vi "ODE-VI-04022016.vi"(0 "Param_Value":dbl[](array[numeric])=[0.35, 180.0, 0.3], 1 "Mod_Value":dbl[](array[numeric]), 3 "Param_IDs":string[](array[string])=["k1", "k2", "compartment"], 4 "Mod_IDs":string[](array[string]), 5 "Initial Conditions for  variables":dbl[](array[numeric])=[0.00015, 0.0], 6 "Simulation Parameters":T4={"Initial Time"=0.0, "Final Time"=100.0, "Time Step"=0.1, "Absolute Tolerance"=0.001, "Relative Tolerance"=1e-06, "Type of Continuous Solver"=enum."Runge-Kutta 45 (variable)", "Discrete Time Step"=2.0, "Minimum Time Step"=1e-06, "Maximum Time Step"=1.0, "Initial Time Step"=0.1} {"Initial Time Step" min=0.0; "Maximum Time Step" min=0.0; "Minimum Time Step" min=0.0; "Discrete Time Step" min=0.0; "Relative Tolerance" min=0.0; "Absolute Tolerance" min=0.0; "Time Step" min=0.0}, 7 "ODE Right Hand Side":string[](array[string])=["-(compartment*k1*a0)+(compartment*k2*a1^2)", "-2*(compartment*k2*a1^2)+2*(compartment*k1*a0)"], 9 "Del Events":bool, 10 "Event Info":T3, 11 "X (name of variables)":string[](array[string])=["a0", "a1"], 12 "All Variables":string[](array[string]), 13 "Rest_Sp_Init_Amnt":string[](array[string])) -> (14 "Concentration vs. Time":cluster{"times":dbl[], dbl[]}[](graph), 19 "Sim Data":cluster{"times":dbl[], "outputs":dbl[][]} {"outputs" format="%#.9g"})   [LabVIEW 2014]
doc: "This example demonstrates how to use the polymorphic ODE solver in both Formula Sting mode and VI mode. Note that VI mode allows the user to set the values of constants via front panel controls, and the formula is implemented as a call by reference to another VI."
uses:
  ODE Simulation Parameters.ctl
  <vilib>/Simulation/Implementation/Shared/SIM Continuous Solvers.ctl
  Event Info.ctl
  <vilib>/Simulation/Utility/Implementation/Shared/SIM Diagram Parameters.ctl
  Stop ODE.vi
  <vilib>/gmath/ode.llb/ODE Solver formula string.vi
  Sim status.vi
  <vilib>/gmath/NI_Gmath.lvlib
panel:
  out "simulation parameters":T1={"Initial Time"=0.0, "Final Time"=10.0, "Time Step"=0.1, "Absolute Tolerance"=0.001, "Relative Tolerance"=0.001, "Continuous Solver"=enum."Runge-Kutta 45 (variable)", "Discrete Time Step"=1.0, "Minimum Time Step"=1e-08, "Maximum Time Step"=1.0, "Initial Time Step"=0.01} {"Initial Time Step" min=0.0; "Maximum Time Step" min=0.0}
  out "error out":errorcluster
  out "transposed array 2":dbl[][](array[numeric])
  out "subarray 2":dbl[](array[numeric])
  out "Array":dbl[][](array[numeric])
  out "transposed array":dbl[][](array[numeric])
  out "Assign Val":string[][](array[string])
  out "Assign Var Idx":i32[][](array[numeric])
  out "Var Idx":i32[](array[numeric])
  out "Math Val":string[](array[string])
  out "Math Op":string[](array[string])
  out "outputs":dbl[][](array[numeric])
  out "subarray":dbl[][](array[numeric])
  out "Flag":i32[](array[numeric])
  out "Delay Val Tot":dbl[](array[numeric])
  out "Delay Val":dbl[](array[numeric])
  out "Delay Val":dbl
  out "Priority":dbl[](array[numeric])
  out "Event Idx":i32
  out "Delay":dbl[](array[numeric])
  out "Total Mods":i32
  out "Time":dbl[](array[numeric])
  out "current data size":i32[](array[numeric])
  # "%"
  # "ds1/dt = - (k1*s1 - k2*s2) \nds2/dt = k1*s1 - k2*s2 - (s2*k2^nL/(k2^nL + s3^nL))\nds4/dt = s2*k2^nL/(k2^nL + s3^nL)\nds5/dt = - (s5 * (krp^nRP/(krp^nRP + s4^nRP))*(kG^nG/ (kG^nG + s6^nG)) - k4*s7)\nds7/dt = (s5 * (krp^nRP/(krp^nRP + s4^nRP))*(kG^nG/ (kG^nG + s6^nG)) - k4*s7) - k4*s7\nds8/dt = k4*s7"
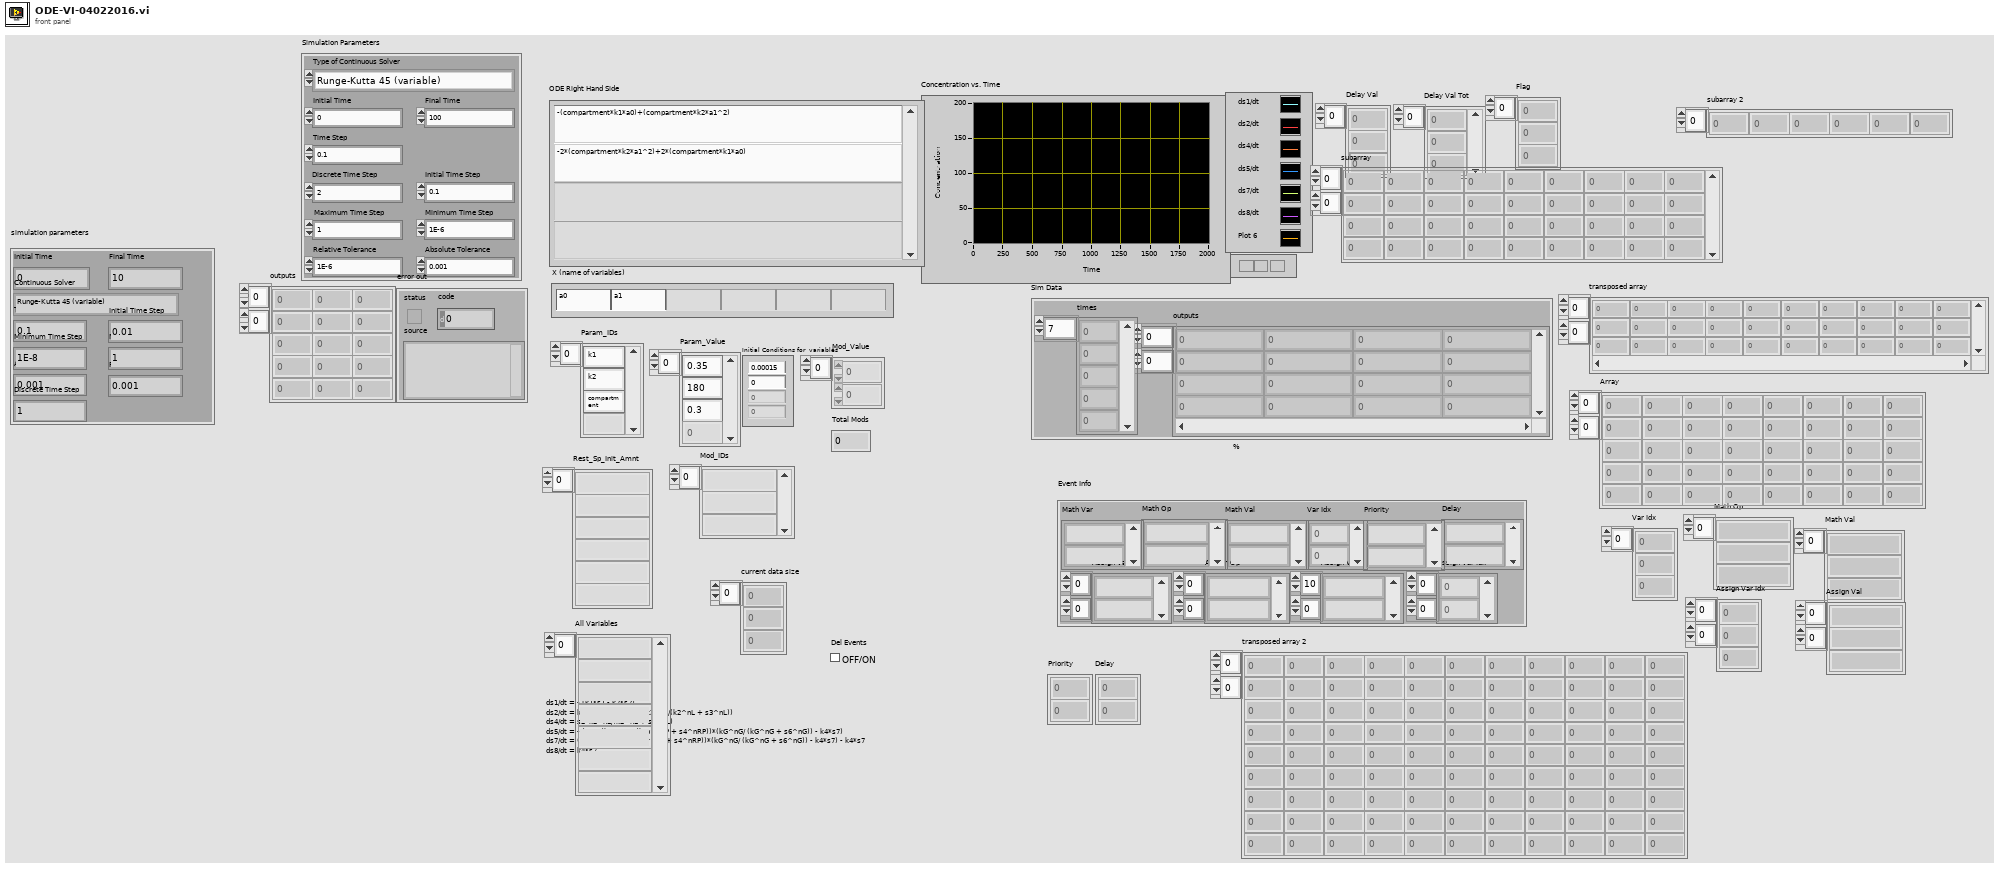
[diagram p1: front panel]
types:
  T1 = typedef "SIM Diagram Parameters.ctl" = cluster{"Initial Time":dbl, "Final Time":dbl, "Time Step":dbl, "Absolute Tolerance":dbl, "Relative Tolerance":dbl, "Continuous Solver":T2, "Discrete Time Step":dbl, "Minimum Time Step":dbl, "Maximum Time Step":dbl, "Initial Time Step":dbl}
  T2 = typedef "SIM Continuous Solvers.ctl" = enum16{"Runge-Kutta 1 (Euler)", "Runge-Kutta 2", "Runge-Kutta 3", "Runge-Kutta 4", "Runge-Kutta 23 (variable)", "Runge-Kutta 45 (variable)", "BDF (variable)", "Adams-Moulton (variable)", "Rosenbrock (variable)", "Discrete States Only"}
  T3 = typedef "Event Info.ctl" = cluster{"Math Var":string[], "Math Op":string[], "Math Val":string[], "Assign Var":string[][], "Assign Op":string[][], "Assign Val":string[][], "Var Idx":i32[], "Assign Var Idx":i32[][], "Delay":string[], "Priority":string[]}
  T4 = typedef "ODE Simulation Parameters.ctl" = cluster{"Initial Time":dbl, "Final Time":dbl, "Time Step":dbl, "Absolute Tolerance":dbl, "Relative Tolerance":dbl, "Type of Continuous Solver":T2, "Discrete Time Step":dbl, "Minimum Time Step":dbl, "Maximum Time Step":dbl, "Initial Time Step":dbl}
  T5 = cluster{"ODE Right Hand Side":string[], "X (name of variables)":string[], "time":string}
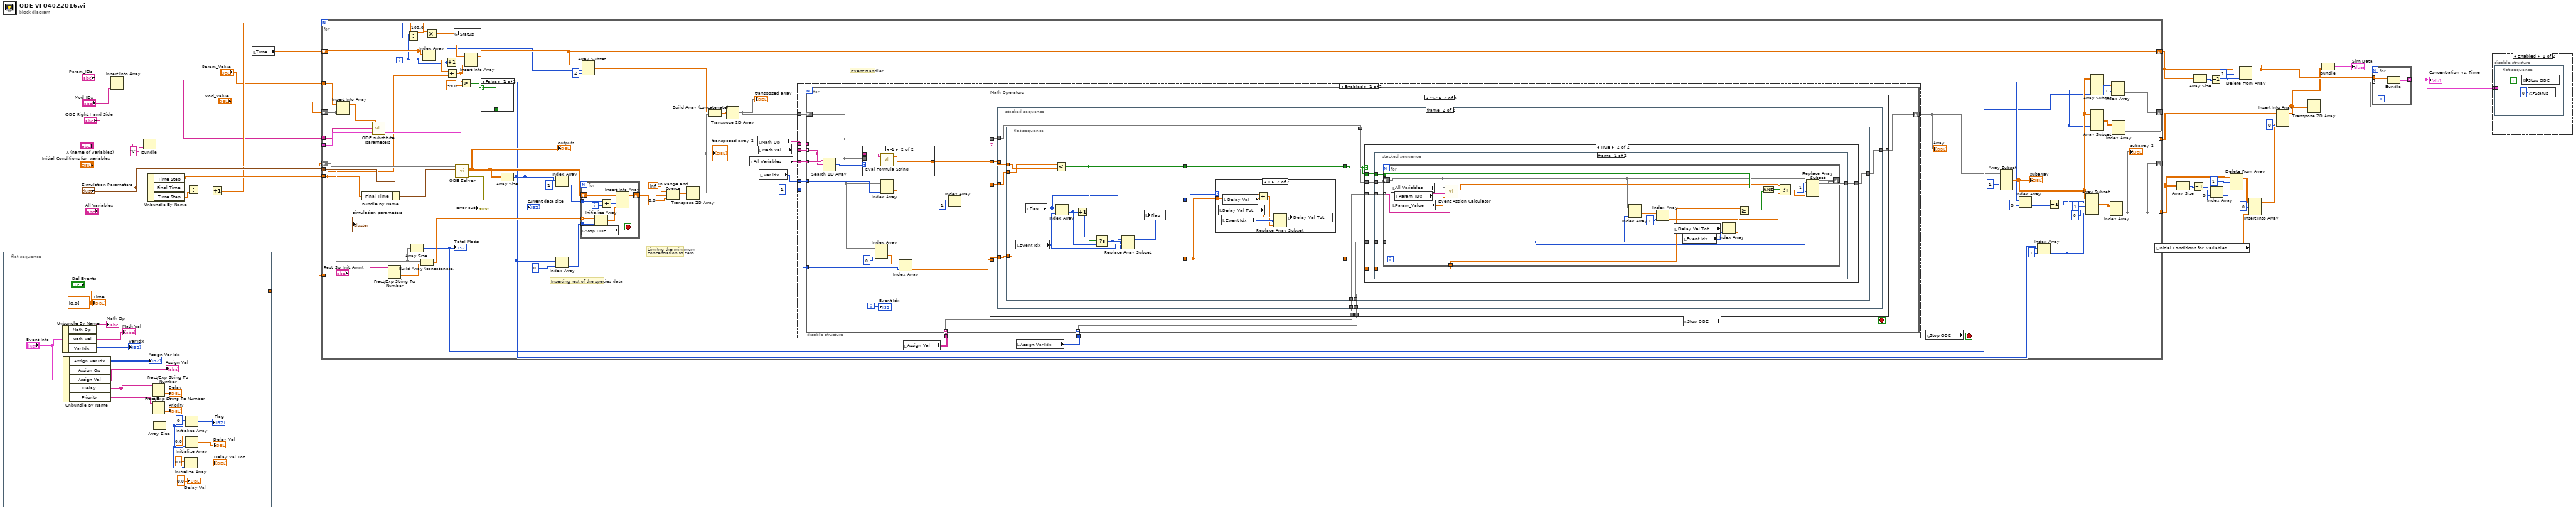
[diagram p0: block diagram]
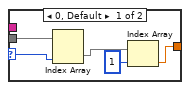
[diagram p4: hidden frame]
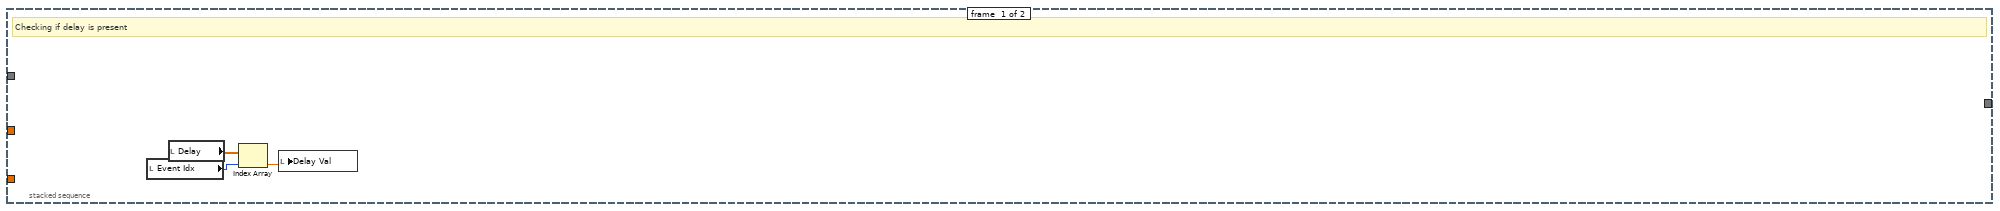
[diagram p6: hidden frame]
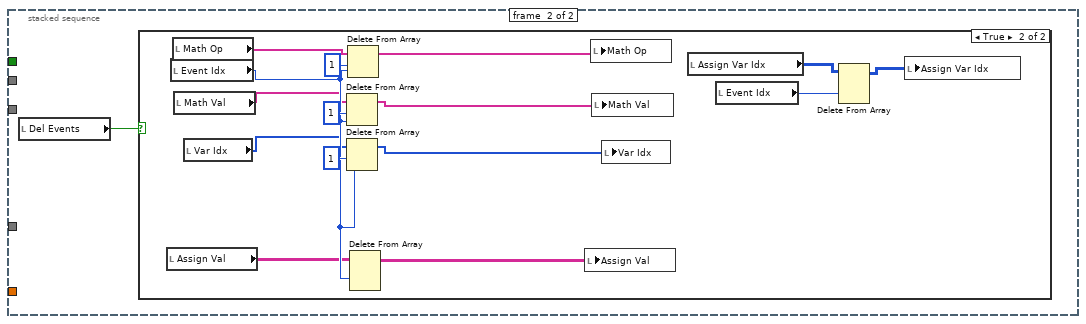
[diagram p9: hidden frame]
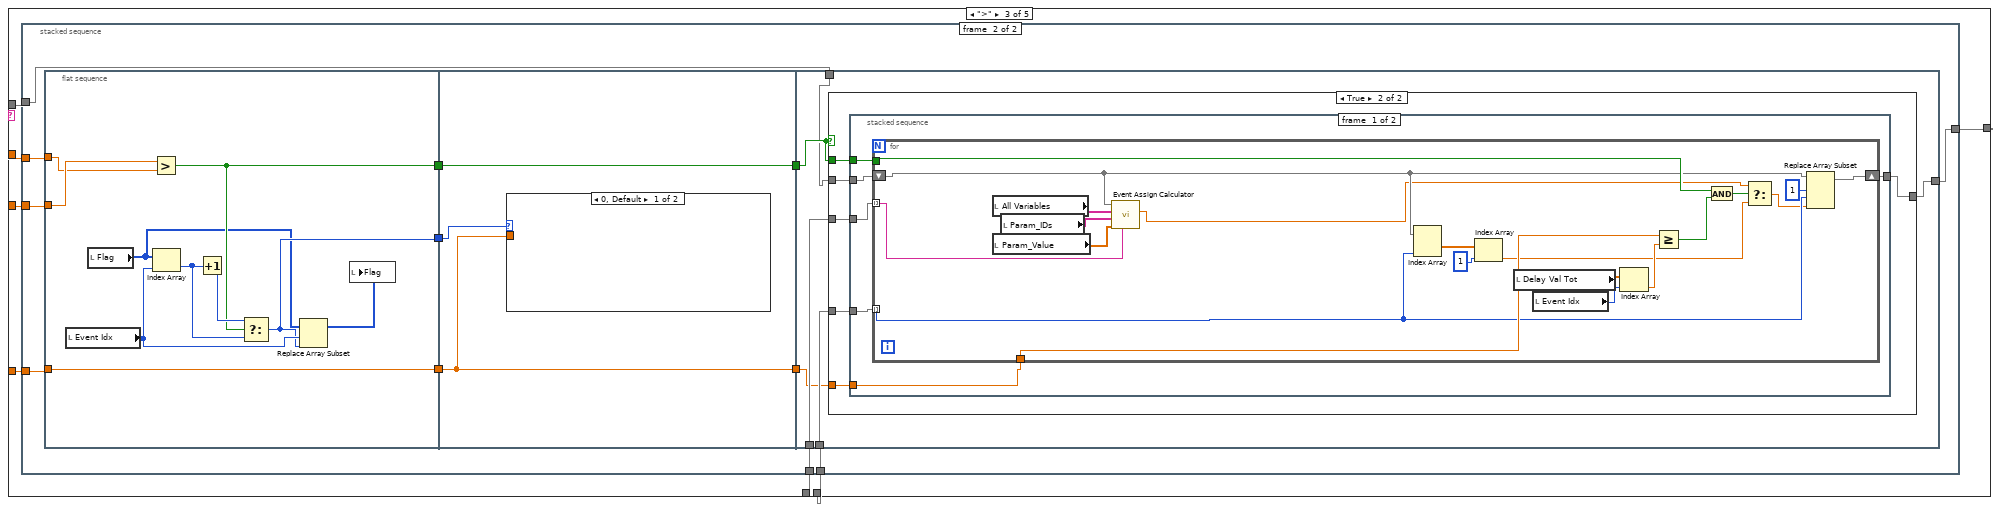
[diagram p11: hidden frame]
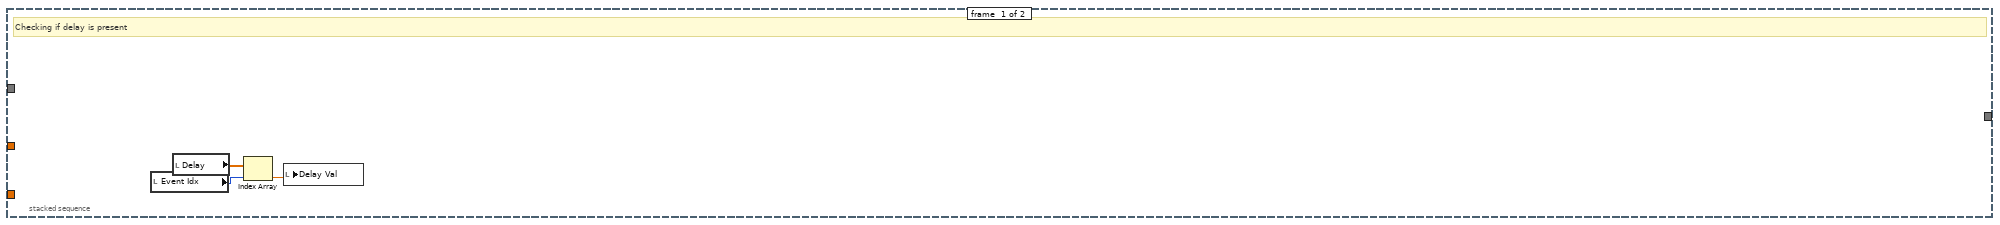
[diagram p12: hidden frame]
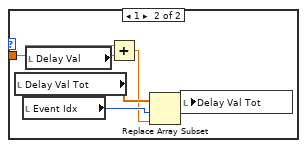
[diagram p13: hidden frame]
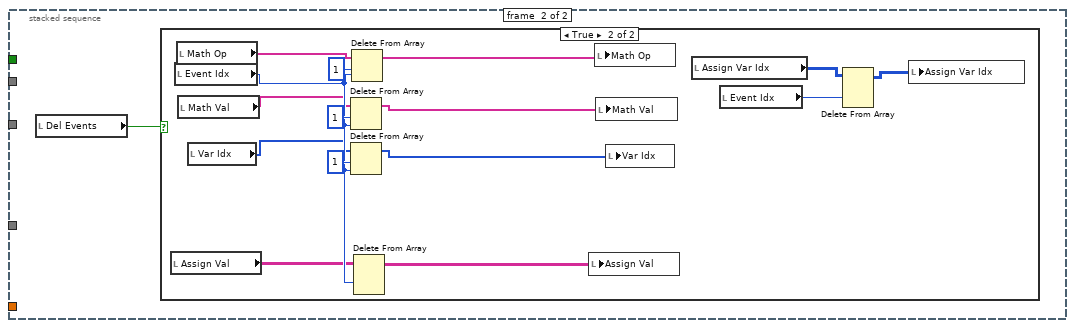
[diagram p15: hidden frame]
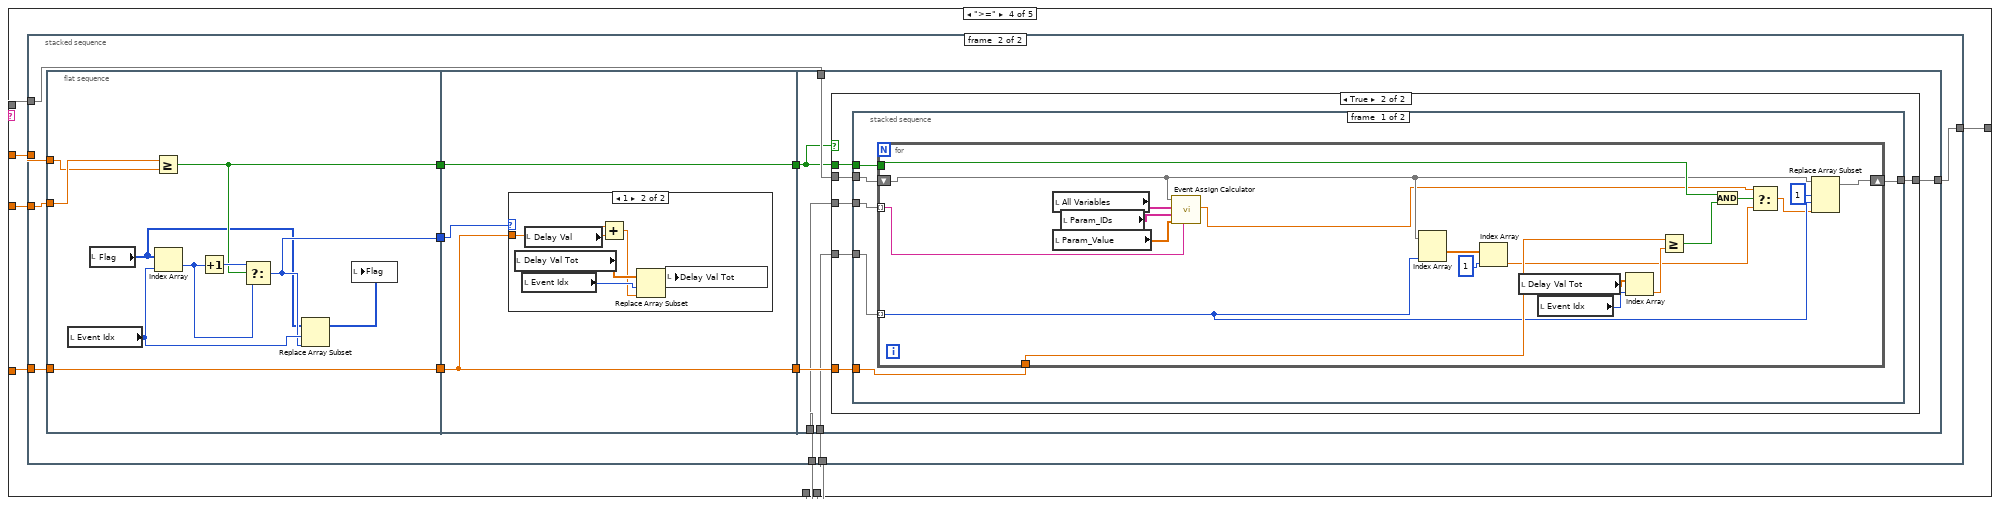
[diagram p17: hidden frame]
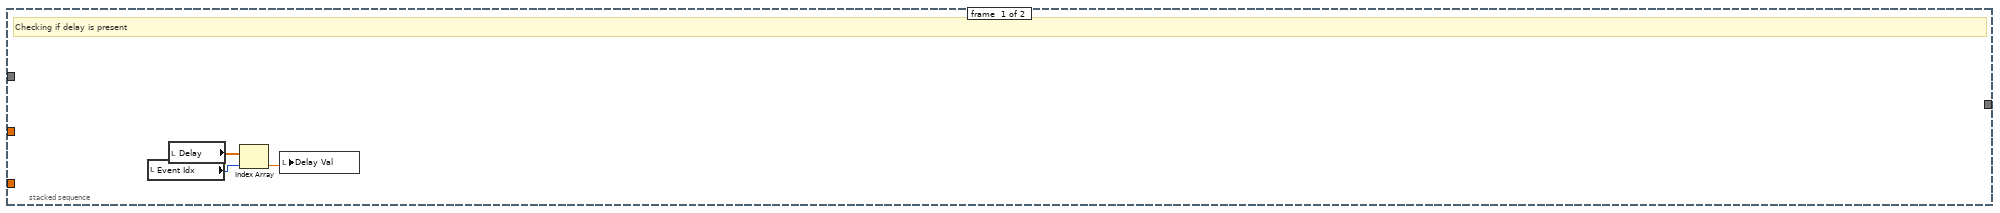
[diagram p18: hidden frame]
diagram:
  n1 = flat-sequence {
    tunnel: [w40] -> w1
    frame #0 {
      w40 = dbl[] [0.0]
      n2 = Unbundle By Name("Event Info") -> ("Math Op"=→"Math Op":string[], "Math Val"=→"Math Val":string[], "Var Idx"=→"Var Idx":i32[])
      n3 = Unbundle By Name("Event Info") -> ("Assign Var Idx"=→"Assign Var Idx":i32[][], "Assign Val"=→"Assign Val":string[][], "Delay"=w49:string[], "Priority"=w52:string[])  [unwired: 1 out]
      n4 = Fract/Exp String To Number(string=w49) -> (number=→"Delay":dbl[])  [unwired: 3 in, 1 out]
      n5 = Fract/Exp String To Number(string=w52) -> (number=→"Priority":dbl[])  [unwired: 3 in, 1 out]
      n6 = Array Size(array=w49) -> (size(s)=w44:i32)
      n7 = Initialize Array(0.0 ("element"), w44) -> (→"Delay Val Tot":dbl[])
      n8 = Initialize Array(0 ("element"), w44) -> (→"Flag":i32[])
      n9 = Initialize Array(0.0 ("element"), w44) -> (→"Delay Val":dbl[])
      "Time" <- w40
      "Delay Val" <- 0.0 ("Delay Val")
    }
  }
  n10 = Insert Into Array(array="Param_IDs", new element="Mod_IDs") -> (w5:string[])  [unwired: 1 in]
  n11 = Bundle("ODE Right Hand Side"="ODE Right Hand Side", "X (name of variables)"="X (name of variables)", "time"="t") -> (w6:T5)  [unwired: 1 in]
  n12 = Unbundle By Name("Simulation Parameters") -> ("Time Step"=w30:dbl, "Final Time"=w32:dbl, "Time Step"=w31:dbl)
  n13 = Divide(x=w32, y=w31) -> (x/y=w28:dbl)
  n14 = Increment(x=w28) -> (x+1=w27:dbl)
  n15 = local read "Time"() -> (w29:dbl[])
  n16 = for {
    N: w27 -> [w74]
    tunnel: "Simulation Parameters" -> [w104]
    shift-right: [w64] -> _
    shift-left: "Initial Conditions for  variables" -> [w125]
    shift-right: [w102] -> w25
    shift-left: w29 -> [w106]
    tunnel: [w64] -> w9 mode=indexing
    tunnel: w30 -> [w59]
    tunnel: [w97] -> w10 mode=indexing
    tunnel: w6 -> [w95]
    tunnel: w5 -> [w94]
    tunnel: "Param_Value" -> [w93]
    shift-right: [w77] -> _
    shift-left: "Mod_Value" -> [w89]
    tunnel: w1 -> [_]
    i -> [w75]
    stop <- w87 stop-if-true
    # "Event Handler"
    # "Limitng the minimum \nconcentration to zero"
    # "Inserting rest of the species data"
    n17 = Insert Into Array(array=w93, new element=w89) -> (w92:dbl[])  [unwired: 1 in]
    n18 = Bundle By Name(cluster=w104, "Final Time"=w59) -> (w103:T4)
    n19 = call "ODE substitute parameters.vi"("Formula String Parameters"=w95, "parameters"=w94, "values"=w92) -> ("Formula String Parameters with substitutions"=w96:T5)  [unwired: 2 out]
    n20 = Fract/Exp String To Number(string="Rest_Sp_Init_Amnt") -> (number=w118:dbl[])  [unwired: 3 in, 1 out]
    n21 = Divide(x=w75, y=w74) -> (x/y=w73:dbl)
    n22 = Array Size(array=w89) -> (size(s)=w88:i32)
    "Total Mods" <- w88
    n23 = Build Array (concatenate)(w89, w118) -> (w117:dbl[])
    n24 = Index Array(array=w106, index=w75) -> (element=w107:dbl)
    n25 = Multiply(x=100.0, y=w73) -> (x*y=w71:dbl)
    n26 = Increment(x=w75) -> (x+1=w105:i32)
    n27 = Add(x=w107, y=w59) -> (x+y=w81:dbl)
    n28 = global write "Sim status.vi" "Status"(w71) -> ()
    n29 = call-poly <vilib>:"ODE Solver.vi"("ODE RHS"=w96, "simulation parameters"=w103, "x0"=w125) -> ("error out"=→"error out":errorcluster, "outputs"=w120:dbl[][])  [unwired: 3 in, 4 out]
    "outputs" <- w120
    n30 = Greater Or Equal?(x=w81, y=99.0) -> (x >= y?=w79:bool)
    n31 = Insert Into Array(array=w106, index=w105, new element=w81) -> (w102:dbl[])
    n32 = case shown="False" w79 {
      selector: w79 -> [w126 w127]
      tunnel: [w126 w127] -> _
      frame False {
      }
      frame True {
      }
    }
    n33 = Array Size(array=w120) -> (size(s)=w99:i32[])
    "current data size" <- w99
    n34 = Index Array(array=w99, index=1) -> (element=w123:i32)
    n35 = Index Array(array=w99, index=0) -> (element=w121:i32)
    n36 = for {
      tunnel: w117 -> [w568] mode=indexing
      tunnel: w123 -> [w570]
      tunnel: w121 -> [w567]
      shift-right: [w564] -> w114
      shift-left: w120 -> [w565]
      i -> [w571]
      stop <- w563 stop-if-true
      n37 = global read "Stop ODE.vi" "Stop ODE"() -> (w563:bool)
      n38 = Initialize Array(w568, w567) -> (w566:dbl[])
      n39 = Add(x=w570, y=w571) -> (x+y=w569:i32)
      n40 = Insert Into Array(array=w565, index (col)=w569, new element=w566) -> (w564:dbl[][])  [unwired: 1 in]
    }
    n41 = Array Subset(array=w102, index=w75, length=2) -> (w100:dbl[])
    n42 = In Range and Coerce(upper limit=inf, x=w114, lower limit=0.0) -> (coerced(x)=w85:dbl[][])  [unwired: 1 out]
    n43 = Transpose 2D Array(2D array=w85) -> (transposed array=w84:dbl[][])
    "transposed array 2" <- w84
    n44 = Build Array (concatenate)(w100, w84) -> (w86:dbl[][])
    n45 = Transpose 2D Array(2D array=w86) -> (transposed array=w83:dbl[][])
    "transposed array" <- w83
    n46 = local read "All Variables"() -> (w65:string[])
    n47 = local read "Math Op"() -> (w70:string[])
    n48 = local read "Math Val"() -> (w69:string[])
    n49 = local read "Var Idx"() -> (w68:i32[])
    n50 = local read "Assign Val"() -> (w66:string[][])
    n51 = local read "Assign Var Idx"() -> (w67:i32[][])
    n52 = disable-structure shown="Enabled" {
      disable-tunnel: w70 -> [w136 w557]
      disable-tunnel: w69 -> [w135 w558]
      disable-tunnel: w68 -> [w134 w559]
      disable-tunnel: w66 -> [w129 w556]
      disable-tunnel: w67 -> [w133 w555]
      disable-tunnel: [w132 w561] -> w63
      disable-tunnel: w83 -> [w131 w562]
      disable-tunnel: 1 ("index") -> [w130 w560]
      disable-tunnel: w65 -> [w128 _]
      frame Enabled {
        n53 = for {
          tunnel: w136 -> [w155] mode=indexing
          tunnel: w135 -> [w139] mode=indexing
          tunnel: w134 -> [w154] mode=indexing
          tunnel: w129 -> [w150] mode=indexing
          tunnel: w133 -> [w153] mode=indexing
          shift-right: [w148] -> w132
          shift-left: w131 -> [w137]
          tunnel: w130 -> [w142]
          tunnel: w128 -> [w140]
          i -> [w151]
          stop <- w152 stop-if-true
          n54 = Search 1D Array(1D array=w140, element=w139) -> (index of element=w138:i32)  [unwired: 1 in]
          n55 = case shown="-1" w138 {
            selector: w138 -> [w159 _]
            tunnel: [w156 w161] -> w149
            tunnel: w139 -> [_ w162]
            tunnel: w137 -> [w160 _]
            frame 0, Default {
              n56 = Index Array(array=w160, index (col)=w159) -> (element=w157:dbl[])  [unwired: 1 in]
              n57 = Index Array(array=w157, index=1) -> (element=w156:dbl)
            }
            frame -1 {
              n58 = call <vilib>:"Eval Formula String.vi"("formula"=w162) -> ("y value"=w161:dbl)  [unwired: 1 in, 1 out]
            }
          }
          n59 = Index Array(array=w137, index (col)=0 ("disabled index (col)")) -> (element=w143:dbl[])  [unwired: 1 in]
          n60 = Index Array(array=w137, index (col)=w154) -> (element=w146:dbl[])  [unwired: 1 in]
          n61 = Index Array(array=w143, index=w142) -> (element=w141:dbl)
          n62 = Index Array(array=w146, index=1) -> (element=w145:dbl)
          n63 = case "Math Operators" shown="\"<\"" w155 {
            tunnel: w149 -> [_ w169 w265 w361 w457]
            tunnel: [w163 w168 w264 w360 w456] -> w148
            tunnel: w137 -> [w163 w170 w266 w362 w458]
            tunnel: w150 -> [_ w167 w263 w359 w455]
            tunnel: w153 -> [_ w166 w262 w358 w454]
            tunnel: w145 -> [_ w165 w261 w356 w453]
            tunnel: w141 -> [_ w164 w260 w357 w452]
            frame "False", Default {
            }
            frame "<" {
              n64 = stacked-sequence {
                tunnel: w169 -> [_ w185]
                tunnel: w170 -> [_ w177]
                tunnel: [_ w176] -> w168
                tunnel: w167 -> [_ w179]
                tunnel: w166 -> [_ w178]
                tunnel: w165 -> [_ w175]
                tunnel: w164 -> [_ w174]
                frame #0 {
                  # "Checking if delay is present"
                  n65 = local read "Event Idx"() -> (w172:i32)
                  n66 = local read "Delay"() -> (w173:dbl[])
                  n67 = Index Array(array=w173, index=w172) -> (element=w171:dbl)
                  n68 = local write "Delay Val"(w171) -> ()
                }
                frame #1 {
                  n69 = flat-sequence {
                    tunnel: w175 -> [w195]
                    tunnel: w185 -> [w194]
                    tunnel: [w189] -> w184
                    tunnel: [w188] -> w183
                    tunnel: [w186] -> w182
                    tunnel: w174 -> [w186]
                    tunnel: w184 -> [w197]
                    tunnel: w183 -> [w198]
                    tunnel: w182 -> [w196]
                    tunnel: [w198] -> w181
                    tunnel: [w196] -> w180
                    tunnel: w181 -> [w210]
                    tunnel: w180 -> [w206]
                    tunnel: w177 -> [w209]
                    tunnel: w178 -> [w207]
                    tunnel: w179 -> [w208]
                    tunnel: [w205] -> w176
                    frame #0 {
                      n70 = local read "Event Idx"() -> (w192:i32)
                      n71 = local read "Flag"() -> (w187:i32[])
                      n72 = Less?(x=w195, y=w194) -> (x < y?=w188:bool)
                      n73 = Index Array(array=w187, index=w192) -> (element=w191:i32)
                      n74 = Increment(x=w191) -> (x+1=w190:i32)
                      n75 = Select(t=w190, s=w188, f=w191) -> (s? t:f=w189:i32)
                      n76 = Replace Array Subset(array=w187, new element=w189, index=w192) -> (w193:i32[])
                      n77 = local write "Flag"(w193) -> ()
                    }
                    frame #1 {
                      n78 = case shown="1" w197 {
                        tunnel: w196 -> [_ w203]
                        frame 0, Default {
                        }
                        frame 1 {
                          n79 = local read "Delay Val Tot"() -> (w202:dbl[])
                          n80 = local read "Event Idx"() -> (w200:i32)
                          n81 = local read "Delay Val"() -> (w204:dbl)
                          n82 = Add(x=w203, y=w204) -> (x+y=w199:dbl)
                          n83 = Replace Array Subset(array=w202, new element=w199, index=w200) -> (w201:dbl[])
                          n84 = local write "Delay Val Tot"(w201) -> ()
                        }
                      }
                    }
                    frame #2 {
                      n85 = case shown="True" w210 {
                        tunnel: w210 -> [_ w217]
                        tunnel: w206 -> [_ w216]
                        tunnel: w209 -> [w211 w215]
                        tunnel: w207 -> [_ w214]
                        tunnel: w208 -> [_ w213]
                        tunnel: [w211 w212] -> w205
                        frame False {
                        }
                        frame True {
                          n86 = stacked-sequence {
                            tunnel: w217 -> [w223 _]
                            tunnel: w216 -> [w222 _]
                            tunnel: w215 -> [w221 _]
                            tunnel: w214 -> [w220 _]
                            tunnel: w213 -> [w219 _]
                            tunnel: [w218 _] -> w212
                            frame #0 {
                              n87 = for {
                                tunnel: w223 -> [w241]
                                tunnel: w222 -> [w240]
                                tunnel: w220 -> [w232] mode=indexing
                                tunnel: w219 -> [w225] mode=indexing
                                shift-right: [w230] -> w218
                                shift-left: w221 -> [w229]
                                n88 = local read "All Variables"() -> (w228:string[])
                                n89 = local read "Param_Value"() -> (w226:dbl[])
                                n90 = local read "Param_IDs"() -> (w227:string[])
                                n91 = call "Event Assign Calculator.vi"("Assign Val"=w225, "Param_Value"=w226, "Param_IDs"=w227, "All Variables"=w228, "transposed array"=w229) -> ("y value"=w224:dbl)  [unwired: 6 in]
                                n92 = Index Array(array=w229, index (col)=w232) -> (element=w235:dbl[])  [unwired: 1 in]
                                n93 = Index Array(array=w235, index=1) -> (element=w234:dbl)
                                n94 = local read "Delay Val Tot"() -> (w239:dbl[])
                                n95 = local read "Event Idx"() -> (w238:i32)
                                n96 = Index Array(array=w239, index=w238) -> (element=w237:dbl)
                                n97 = Greater Or Equal?(x=w240, y=w237) -> (x >= y?=w242:bool)
                                n98 = And(x=w241, y=w242) -> (x .and. y?=w243:bool)
                                n99 = Select(t=w224, s=w243, f=w234) -> (s? t:f=w231:dbl)
                                n100 = Replace Array Subset(array=w229, new element=w231, index (row)=1, index (col)=w232) -> (w230:dbl[][])
                              }
                            }
                            frame #1 {
                              n101 = local read "Del Events"() -> (w244:bool)
                              n102 = case shown="True" w244 {
                                frame False {
                                }
                                frame True {
                                n103 = local read "Assign Val"() -> (w249:string[][])
                                n104 = local read "Event Idx"() -> (w256:i32)
                                n105 = local read "Math Op"() -> (w255:string[])
                                n106 = local read "Math Val"() -> (w254:string[])
                                n107 = local read "Var Idx"() -> (w253:i32[])
                                n108 = Delete From Array(array=w254, length=1, index=w256) -> (array with subset deleted=w251:string[])  [unwired: 1 out]
                                n109 = Delete From Array(array=w253, length=1, index=w256) -> (array with subset deleted=w250:i32[])  [unwired: 1 out]
                                n110 = Delete From Array(array=w255, length=1, index=w256) -> (array with subset deleted=w252:string[])  [unwired: 1 out]
                                n111 = Delete From Array(array=w249, index (row)=w256) -> (array with subset deleted=w248:string[][])  [unwired: 2 in, 1 out]
                                n112 = local write "Assign Val"(w248) -> ()
                                n113 = local write "Math Op"(w252) -> ()
                                n114 = local write "Math Val"(w251) -> ()
                                n115 = local write "Var Idx"(w250) -> ()
                                n116 = local read "Assign Var Idx"() -> (w247:i32[][])
                                n117 = local read "Event Idx"() -> (w246:i32)
                                n118 = Delete From Array(array=w247, index (row)=w246) -> (array with subset deleted=w245:i32[][])  [unwired: 2 in, 1 out]
                                n119 = local write "Assign Var Idx"(w245) -> ()
                                }
                              }
                            }
                          }
                        }
                      }
                    }
                  }
                }
              }
            }
            frame ">" {
              n120 = stacked-sequence {
                tunnel: w265 -> [_ w281]
                tunnel: w266 -> [_ w273]
                tunnel: [_ w272] -> w264
                tunnel: w263 -> [_ w275]
                tunnel: w262 -> [_ w274]
                tunnel: w261 -> [_ w271]
                tunnel: w260 -> [_ w270]
                frame #0 {
                  # "Checking if delay is present"
                  n121 = local read "Event Idx"() -> (w268:i32)
                  n122 = local read "Delay"() -> (w269:dbl[])
                  n123 = Index Array(array=w269, index=w268) -> (element=w267:dbl)
                  n124 = local write "Delay Val"(w267) -> ()
                }
                frame #1 {
                  n125 = flat-sequence {
                    tunnel: w271 -> [w291]
                    tunnel: w281 -> [w290]
                    tunnel: w270 -> [w289]
                    tunnel: [w284] -> w280
                    tunnel: [w283] -> w279
                    tunnel: [w289] -> w278
                    tunnel: w280 -> [w293]
                    tunnel: w279 -> [w294]
                    tunnel: w278 -> [w292]
                    tunnel: [w294] -> w277
                    tunnel: [w292] -> w276
                    tunnel: w277 -> [w306]
                    tunnel: w276 -> [w302]
                    tunnel: w273 -> [w305]
                    tunnel: w274 -> [w303]
                    tunnel: w275 -> [w304]
                    tunnel: [w301] -> w272
                    frame #0 {
                      n126 = local read "Event Idx"() -> (w287:i32)
                      n127 = local read "Flag"() -> (w282:i32[])
                      n128 = Greater?(x=w291, y=w290) -> (0:w283:bool)
                      n129 = Index Array(array=w282, index=w287) -> (element=w286:i32)
                      n130 = Increment(x=w286) -> (x+1=w285:i32)
                      n131 = Select(t=w285, s=w283, f=w286) -> (s? t:f=w284:i32)
                      n132 = Replace Array Subset(array=w282, new element=w284, index=w287) -> (w288:i32[])
                      n133 = local write "Flag"(w288) -> ()
                    }
                    frame #1 {
                      n134 = case shown="0, Default" w293 {
                        tunnel: w292 -> [_ w299]
                        frame 0, Default {
                        }
                        frame 1 {
                          n135 = local read "Delay Val Tot"() -> (w298:dbl[])
                          n136 = local read "Event Idx"() -> (w296:i32)
                          n137 = local read "Delay Val"() -> (w300:dbl)
                          n138 = Add(x=w299, y=w300) -> (x+y=w295:dbl)
                          n139 = Replace Array Subset(array=w298, new element=w295, index=w296) -> (w297:dbl[])
                          n140 = local write "Delay Val Tot"(w297) -> ()
                        }
                      }
                    }
                    frame #2 {
                      n141 = case shown="True" w306 {
                        tunnel: w306 -> [_ w313]
                        tunnel: w302 -> [_ w312]
                        tunnel: w305 -> [w307 w311]
                        tunnel: w303 -> [_ w310]
                        tunnel: w304 -> [_ w309]
                        tunnel: [w307 w308] -> w301
                        frame False {
                        }
                        frame True {
                          n142 = stacked-sequence {
                            tunnel: w313 -> [w317 _]
                            tunnel: w312 -> [w314 _]
                            tunnel: w311 -> [w316 _]
                            tunnel: w310 -> [w318 _]
                            tunnel: w309 -> [w315 _]
                            tunnel: [w319 _] -> w308
                            frame #0 {
                              n143 = for {
                                tunnel: w317 -> [w337]
                                tunnel: w314 -> [w336]
                                tunnel: w318 -> [w328] mode=indexing
                                tunnel: w315 -> [w322] mode=indexing
                                shift-right: [w326] -> w319
                                shift-left: w316 -> [w321]
                                n144 = local read "All Variables"() -> (w325:string[])
                                n145 = local read "Param_Value"() -> (w323:dbl[])
                                n146 = local read "Param_IDs"() -> (w324:string[])
                                n147 = call "Event Assign Calculator.vi"("Assign Val"=w322, "Param_Value"=w323, "Param_IDs"=w324, "All Variables"=w325, "transposed array"=w321) -> ("y value"=w320:dbl)  [unwired: 6 in]
                                n148 = Index Array(array=w321, index (col)=w328) -> (element=w331:dbl[])  [unwired: 1 in]
                                n149 = Index Array(array=w331, index=1) -> (element=w330:dbl)
                                n150 = local read "Delay Val Tot"() -> (w335:dbl[])
                                n151 = local read "Event Idx"() -> (w334:i32)
                                n152 = Index Array(array=w335, index=w334) -> (element=w333:dbl)
                                n153 = Greater Or Equal?(x=w336, y=w333) -> (x >= y?=w338:bool)
                                n154 = And(x=w337, y=w338) -> (x .and. y?=w339:bool)
                                n155 = Select(t=w320, s=w339, f=w330) -> (s? t:f=w327:dbl)
                                n156 = Replace Array Subset(array=w321, new element=w327, index (row)=1, index (col)=w328) -> (w326:dbl[][])
                              }
                            }
                            frame #1 {
                              n157 = local read "Del Events"() -> (w340:bool)
                              n158 = case shown="True" w340 {
                                frame False {
                                }
                                frame True {
                                n159 = local read "Assign Val"() -> (w345:string[][])
                                n160 = local read "Event Idx"() -> (w352:i32)
                                n161 = local read "Math Op"() -> (w351:string[])
                                n162 = local read "Math Val"() -> (w350:string[])
                                n163 = local read "Var Idx"() -> (w349:i32[])
                                n164 = Delete From Array(array=w350, length=1, index=w352) -> (array with subset deleted=w347:string[])  [unwired: 1 out]
                                n165 = Delete From Array(array=w349, length=1, index=w352) -> (array with subset deleted=w346:i32[])  [unwired: 1 out]
                                n166 = Delete From Array(array=w351, length=1, index=w352) -> (array with subset deleted=w348:string[])  [unwired: 1 out]
                                n167 = Delete From Array(array=w345, index (row)=w352) -> (array with subset deleted=w344:string[][])  [unwired: 2 in, 1 out]
                                n168 = local write "Assign Val"(w344) -> ()
                                n169 = local write "Math Op"(w348) -> ()
                                n170 = local write "Math Val"(w347) -> ()
                                n171 = local write "Var Idx"(w346) -> ()
                                n172 = local read "Assign Var Idx"() -> (w343:i32[][])
                                n173 = local read "Event Idx"() -> (w342:i32)
                                n174 = Delete From Array(array=w343, index (row)=w342) -> (array with subset deleted=w341:i32[][])  [unwired: 2 in, 1 out]
                                n175 = local write "Assign Var Idx"(w341) -> ()
                                }
                              }
                            }
                          }
                        }
                      }
                    }
                  }
                }
              }
            }
            frame ">=" {
              n176 = stacked-sequence {
                tunnel: w361 -> [_ w377]
                tunnel: w362 -> [_ w369]
                tunnel: [_ w368] -> w360
                tunnel: w359 -> [_ w371]
                tunnel: w358 -> [_ w370]
                tunnel: w357 -> [_ w367]
                tunnel: w356 -> [_ w366]
                frame #0 {
                  # "Checking if delay is present"
                  n177 = local read "Event Idx"() -> (w364:i32)
                  n178 = local read "Delay"() -> (w365:dbl[])
                  n179 = Index Array(array=w365, index=w364) -> (element=w363:dbl)
                  n180 = local write "Delay Val"(w363) -> ()
                }
                frame #1 {
                  n181 = flat-sequence {
                    tunnel: w366 -> [w387]
                    tunnel: w377 -> [w386]
                    tunnel: w367 -> [w385]
                    tunnel: [w380] -> w376
                    tunnel: [w379] -> w375
                    tunnel: [w385] -> w374
                    tunnel: w376 -> [w389]
                    tunnel: w375 -> [w390]
                    tunnel: w374 -> [w388]
                    tunnel: [w390] -> w373
                    tunnel: [w388] -> w372
                    tunnel: w373 -> [w397]
                    tunnel: w372 -> [w402]
                    tunnel: w369 -> [w401]
                    tunnel: w370 -> [w400]
                    tunnel: w371 -> [w399]
                    tunnel: [w398] -> w368
                    frame #0 {
                      n182 = local read "Event Idx"() -> (w383:i32)
                      n183 = local read "Flag"() -> (w378:i32[])
                      n184 = Greater Or Equal?(x=w387, y=w386) -> (x >= y?=w379:bool)
                      n185 = Index Array(array=w378, index=w383) -> (element=w382:i32)
                      n186 = Increment(x=w382) -> (x+1=w381:i32)
                      n187 = Select(t=w381, s=w379, f=w382) -> (s? t:f=w380:i32)
                      n188 = Replace Array Subset(array=w378, new element=w380, index=w383) -> (w384:i32[])
                      n189 = local write "Flag"(w384) -> ()
                    }
                    frame #1 {
                      n190 = case shown="1" w389 {
                        tunnel: w388 -> [_ w395]
                        frame 0, Default {
                        }
                        frame 1 {
                          n191 = local read "Delay Val Tot"() -> (w394:dbl[])
                          n192 = local read "Event Idx"() -> (w392:i32)
                          n193 = local read "Delay Val"() -> (w396:dbl)
                          n194 = Add(x=w395, y=w396) -> (x+y=w391:dbl)
                          n195 = Replace Array Subset(array=w394, new element=w391, index=w392) -> (w393:dbl[])
                          n196 = local write "Delay Val Tot"(w393) -> ()
                        }
                      }
                    }
                    frame #2 {
                      n197 = case shown="True" w397 {
                        tunnel: w397 -> [_ w409]
                        tunnel: w402 -> [_ w408]
                        tunnel: w401 -> [w403 w407]
                        tunnel: w400 -> [_ w406]
                        tunnel: w399 -> [_ w405]
                        tunnel: [w403 w404] -> w398
                        frame False {
                        }
                        frame True {
                          n198 = stacked-sequence {
                            tunnel: w409 -> [w414 _]
                            tunnel: w408 -> [w411 _]
                            tunnel: w407 -> [w415 _]
                            tunnel: w406 -> [w412 _]
                            tunnel: w405 -> [w413 _]
                            tunnel: [w410 _] -> w404
                            frame #0 {
                              n199 = for {
                                tunnel: w414 -> [w433]
                                tunnel: w411 -> [w432]
                                tunnel: w412 -> [w424] mode=indexing
                                tunnel: w413 -> [w418] mode=indexing
                                shift-right: [w422] -> w410
                                shift-left: w415 -> [w417]
                                n200 = local read "All Variables"() -> (w421:string[])
                                n201 = local read "Param_Value"() -> (w419:dbl[])
                                n202 = local read "Param_IDs"() -> (w420:string[])
                                n203 = call "Event Assign Calculator.vi"("Assign Val"=w418, "Param_Value"=w419, "Param_IDs"=w420, "All Variables"=w421, "transposed array"=w417) -> ("y value"=w416:dbl)  [unwired: 6 in]
                                n204 = Index Array(array=w417, index (col)=w424) -> (element=w427:dbl[])  [unwired: 1 in]
                                n205 = Index Array(array=w427, index=1) -> (element=w426:dbl)
                                n206 = local read "Delay Val Tot"() -> (w431:dbl[])
                                n207 = local read "Event Idx"() -> (w430:i32)
                                n208 = Index Array(array=w431, index=w430) -> (element=w429:dbl)
                                n209 = Greater Or Equal?(x=w432, y=w429) -> (x >= y?=w434:bool)
                                n210 = And(x=w433, y=w434) -> (x .and. y?=w435:bool)
                                n211 = Select(t=w416, s=w435, f=w426) -> (s? t:f=w423:dbl)
                                n212 = Replace Array Subset(array=w417, new element=w423, index (row)=1, index (col)=w424) -> (w422:dbl[][])
                              }
                            }
                            frame #1 {
                              n213 = local read "Del Events"() -> (w436:bool)
                              n214 = case shown="True" w436 {
                                frame False {
                                }
                                frame True {
                                n215 = local read "Assign Val"() -> (w441:string[][])
                                n216 = local read "Event Idx"() -> (w448:i32)
                                n217 = local read "Math Op"() -> (w447:string[])
                                n218 = local read "Math Val"() -> (w446:string[])
                                n219 = local read "Var Idx"() -> (w445:i32[])
                                n220 = Delete From Array(array=w446, length=1, index=w448) -> (array with subset deleted=w443:string[])  [unwired: 1 out]
                                n221 = Delete From Array(array=w445, length=1, index=w448) -> (array with subset deleted=w442:i32[])  [unwired: 1 out]
                                n222 = Delete From Array(array=w447, length=1, index=w448) -> (array with subset deleted=w444:string[])  [unwired: 1 out]
                                n223 = Delete From Array(array=w441, index (row)=w448) -> (array with subset deleted=w440:string[][])  [unwired: 2 in, 1 out]
                                n224 = local write "Assign Val"(w440) -> ()
                                n225 = local write "Math Op"(w444) -> ()
                                n226 = local write "Math Val"(w443) -> ()
                                n227 = local write "Var Idx"(w442) -> ()
                                n228 = local read "Assign Var Idx"() -> (w439:i32[][])
                                n229 = local read "Event Idx"() -> (w438:i32)
                                n230 = Delete From Array(array=w439, index (row)=w438) -> (array with subset deleted=w437:i32[][])  [unwired: 2 in, 1 out]
                                n231 = local write "Assign Var Idx"(w437) -> ()
                                }
                              }
                            }
                          }
                        }
                      }
                    }
                  }
                }
              }
            }
            frame "<=" {
              n232 = stacked-sequence {
                tunnel: w457 -> [_ w473]
                tunnel: w458 -> [_ w465]
                tunnel: [_ w462] -> w456
                tunnel: w455 -> [_ w467]
                tunnel: w454 -> [_ w466]
                tunnel: w453 -> [_ w464]
                tunnel: w452 -> [_ w463]
                frame #0 {
                  # "Checking if delay is present"
                  n233 = local read "Event Idx"() -> (w460:i32)
                  n234 = local read "Delay"() -> (w461:dbl[])
                  n235 = Index Array(array=w461, index=w460) -> (element=w459:dbl)
                  n236 = local write "Delay Val"(w459) -> ()
                }
                frame #1 {
                  n237 = flat-sequence {
                    tunnel: w464 -> [w483]
                    tunnel: w473 -> [w482]
                    tunnel: w463 -> [w481]
                    tunnel: [w476] -> w472
                    tunnel: [w475] -> w471
                    tunnel: [w481] -> w470
                    tunnel: w472 -> [w485]
                    tunnel: w471 -> [w486]
                    tunnel: w470 -> [w484]
                    tunnel: [w486] -> w469
                    tunnel: [w484] -> w468
                    tunnel: w469 -> [w498]
                    tunnel: w468 -> [w494]
                    tunnel: w465 -> [w497]
                    tunnel: w466 -> [w495]
                    tunnel: w467 -> [w496]
                    tunnel: [w493] -> w462
                    frame #0 {
                      n238 = local read "Event Idx"() -> (w479:i32)
                      n239 = local read "Flag"() -> (w474:i32[])
                      n240 = Less Or Equal?(x=w483, y=w482) -> (x <= y?=w475:bool)
                      n241 = Index Array(array=w474, index=w479) -> (element=w478:i32)
                      n242 = Increment(x=w478) -> (x+1=w477:i32)
                      n243 = Select(t=w477, s=w475, f=w478) -> (s? t:f=w476:i32)
                      n244 = Replace Array Subset(array=w474, new element=w476, index=w479) -> (w480:i32[])
                      n245 = local write "Flag"(w480) -> ()
                    }
                    frame #1 {
                      n246 = case shown="1" w485 {
                        tunnel: w484 -> [_ w491]
                        frame 0, Default {
                        }
                        frame 1 {
                          n247 = local read "Delay Val Tot"() -> (w490:dbl[])
                          n248 = local read "Event Idx"() -> (w488:i32)
                          n249 = local read "Delay Val"() -> (w492:dbl)
                          n250 = Add(x=w491, y=w492) -> (x+y=w487:dbl)
                          n251 = Replace Array Subset(array=w490, new element=w487, index=w488) -> (w489:dbl[])
                          n252 = local write "Delay Val Tot"(w489) -> ()
                        }
                      }
                    }
                    frame #2 {
                      n253 = case shown="True" w498 {
                        tunnel: w498 -> [_ w505]
                        tunnel: w494 -> [_ w504]
                        tunnel: w497 -> [w499 w503]
                        tunnel: w495 -> [_ w502]
                        tunnel: w496 -> [_ w501]
                        tunnel: [w499 w500] -> w493
                        frame False {
                        }
                        frame True {
                          n254 = stacked-sequence {
                            tunnel: w505 -> [w511 _]
                            tunnel: w504 -> [w507 _]
                            tunnel: w503 -> [w510 _]
                            tunnel: w502 -> [w508 _]
                            tunnel: w501 -> [w509 _]
                            tunnel: [w506 _] -> w500
                            frame #0 {
                              n255 = for {
                                tunnel: w511 -> [w529]
                                tunnel: w507 -> [w528]
                                tunnel: w508 -> [w520] mode=indexing
                                tunnel: w509 -> [w514] mode=indexing
                                shift-right: [w518] -> w506
                                shift-left: w510 -> [w513]
                                n256 = local read "All Variables"() -> (w517:string[])
                                n257 = local read "Param_Value"() -> (w515:dbl[])
                                n258 = local read "Param_IDs"() -> (w516:string[])
                                n259 = call "Event Assign Calculator.vi"("Assign Val"=w514, "Param_Value"=w515, "Param_IDs"=w516, "All Variables"=w517, "transposed array"=w513) -> ("y value"=w512:dbl)  [unwired: 6 in]
                                n260 = Index Array(array=w513, index (col)=w520) -> (element=w523:dbl[])  [unwired: 1 in]
                                n261 = Index Array(array=w523, index=1) -> (element=w522:dbl)
                                n262 = local read "Delay Val Tot"() -> (w527:dbl[])
                                n263 = local read "Event Idx"() -> (w526:i32)
                                n264 = Index Array(array=w527, index=w526) -> (element=w525:dbl)
                                n265 = Greater Or Equal?(x=w528, y=w525) -> (x >= y?=w530:bool)
                                n266 = And(x=w529, y=w530) -> (x .and. y?=w531:bool)
                                n267 = Select(t=w512, s=w531, f=w522) -> (s? t:f=w519:dbl)
                                n268 = Replace Array Subset(array=w513, new element=w519, index (row)=1, index (col)=w520) -> (w518:dbl[][])
                              }
                            }
                            frame #1 {
                              n269 = local read "Del Events"() -> (w532:bool)
                              n270 = case shown="True" w532 {
                                frame False {
                                }
                                frame True {
                                n271 = local read "Assign Val"() -> (w537:string[][])
                                n272 = local read "Event Idx"() -> (w544:i32)
                                n273 = local read "Math Op"() -> (w543:string[])
                                n274 = local read "Math Val"() -> (w542:string[])
                                n275 = local read "Var Idx"() -> (w541:i32[])
                                n276 = Delete From Array(array=w542, length=1, index=w544) -> (array with subset deleted=w539:string[])  [unwired: 1 out]
                                n277 = Delete From Array(array=w541, length=1, index=w544) -> (array with subset deleted=w538:i32[])  [unwired: 1 out]
                                n278 = Delete From Array(array=w543, length=1, index=w544) -> (array with subset deleted=w540:string[])  [unwired: 1 out]
                                n279 = Delete From Array(array=w537, index (row)=w544) -> (array with subset deleted=w536:string[][])  [unwired: 2 in, 1 out]
                                n280 = local write "Assign Val"(w536) -> ()
                                n281 = local write "Math Op"(w540) -> ()
                                n282 = local write "Math Val"(w539) -> ()
                                n283 = local write "Var Idx"(w538) -> ()
                                n284 = local read "Assign Var Idx"() -> (w535:i32[][])
                                n285 = local read "Event Idx"() -> (w534:i32)
                                n286 = Delete From Array(array=w535, index (row)=w534) -> (array with subset deleted=w533:i32[][])  [unwired: 2 in, 1 out]
                                n287 = local write "Assign Var Idx"(w533) -> ()
                                }
                              }
                            }
                          }
                        }
                      }
                    }
                  }
                }
              }
            }
          }
          n288 = global read "Stop ODE.vi" "Stop ODE"() -> (w152:bool)
          "Event Idx" <- w151
        }
      }
      frame Disabled {
        n289 = local read "Delay Val Tot"() -> (w550:dbl[])
        n290 = local read "Delay"() -> (w552:dbl[])
        n291 = local read "Flag"() -> (w551:i32[])
        n292 = local read "Delay Val"() -> (w553:dbl)
        n293 = local read "Priority"() -> (w554:dbl[])
        n294 = call "SBML Events Handler.vi"("Sim Data w/ time"=w562, "Math Op"=w557, "Math Val"=w558, "Var Idx"=w559, "Idx of Time"=w560, "Assign Val"=w556, "Delay"=w552, "Assign Var Idx"=w555, "Flag"=w551, "Priority"=w554, "Delay Val Tot"=w550, "Delay Val"=w553) -> ("Output Data"=w561:dbl[][], "Flag Out"=w549:i32[], "Delay Val Tot Out"=w548:dbl[])  [unwired: 5 in]
        n295 = local write "Delay Val Tot"(w548) -> ()
        n296 = local write "Flag"(w549) -> ()
      }
    }
    "Array" <- w63
    n297 = global read "Stop ODE.vi" "Stop ODE"() -> (w87:bool)
    n298 = Array Subset(array=w63, index (col)=1 ("index (row)")) -> (w91:dbl[][])  [unwired: 3 in]
    "subarray" <- w91
    n299 = Index Array(array=w99, index=0) -> (element=w61:i32)
    n300 = Index Array(array=w99, index=1) -> (element=w90:i32)
    n301 = Decrement(x=w61) -> (x-1=w62:i32)
    n302 = Array Subset(array=w91, index (row)=w62, length (row)=1 ("length"), index (col)=0 ("length"), length (col)=w90) -> (w108:dbl[][])
    n303 = Array Subset(array=w91, index (col)=w90, length (col)=w88) -> (w78:dbl[][])  [unwired: 2 in]
    n304 = Array Subset(array=w91, index (col)=w90) -> (w98:dbl[][])  [unwired: 3 in]
    n305 = Index Array(array=w108) -> (element=w64:dbl[])  [unwired: 2 in]
    "subarray 2" <- w64
    n306 = Index Array(array=w78, index (row)=1) -> (element=w77:dbl[])  [unwired: 1 in]
    n307 = Index Array(array=w98) -> (element=w97:dbl[])  [unwired: 2 in]
  }
  n308 = local read "Initial Conditions for  variables"() -> (w20:dbl[])
  n309 = Array Size(array=w9) -> (size(s)=w17:i32[])
  n310 = Decrement(x=w17) -> (x-1=w15:i32[])
  n311 = Array Size(array=w25) -> (size(s)=w23:i32)
  n312 = Decrement(x=w23) -> (x-1=w22:i32)
  n313 = Index Array(array=w15, index=0) -> (element=w13:i32)
  n314 = Delete From Array(array=w9, length=1, index (row)=w13) -> (array with subset deleted=w12:dbl[][])  [unwired: 1 in, 1 out]
  n315 = Delete From Array(array=w25, length=1, index=w22) -> (array with subset deleted=w18:dbl[])  [unwired: 1 out]
  n316 = Insert Into Array(array=w12, index (row)=0, new element=w20) -> (w8:dbl[][])  [unwired: 1 in]
  n317 = Insert Into Array(array=w10, index (col)=0 ("disabled index (col)"), new element=w8) -> (w7:dbl[][])  [unwired: 1 in]
  n318 = Transpose 2D Array(2D array=w7) -> (transposed array=w21:dbl[][])
  n319 = Bundle("Time"=w18, w7) -> (→"Sim Data":cluster{"Time":dbl[], dbl[][]})  [unwired: 1 in]
  n320 = for {
    tunnel: w18 -> [w573]
    tunnel: [w574] -> w2 mode=indexing
    tunnel: w21 -> [w572] mode=indexing
    n321 = Bundle("Time"=w573, w572) -> (w574:cluster{"Time":dbl[], dbl[]})  [unwired: 1 out]
  }
  "Concentration vs. Time" <- w2
  n322 = disable-structure shown="Enabled" {
    disable-tunnel: w2 -> [w575 _]
    frame Enabled {
      n323 = flat-sequence {
        tunnel: w575 -> [_]
        frame #0 {
          n324 = global write "Stop ODE.vi" "Stop ODE"(TRUE) -> ()
          n325 = global write "Sim status.vi" "Status"(0 ("Status")) -> ()
        }
      }
    }
    frame Disabled {
    }
  }
